vi "fgv_DO_q.vi"(7 "cmd":T1, 8 "error in":errorcluster, 11 "data":T2=enum."start") -> (0 "error out":errorcluster, 3 "queue out":refnum<queue>)   [LabVIEW 2019]
uses:
  _ctrl/start.ctl
  _ctrl/create-rw-close.ctl
  Durability/common/UI.ctl
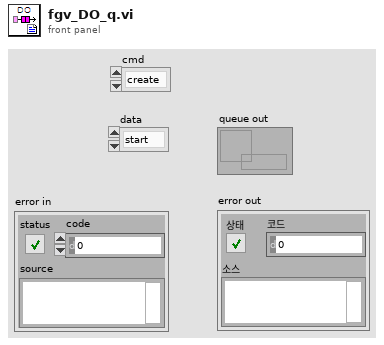
[diagram p1: front panel]
types:
  T1 = typedef "create-rw-close.ctl" = enum16{"create", "write", "read", "delete", "close"}
  T2 = typedef "start.ctl" = enum16{"init", "open", "set", "start", "stop", "read", "read_items", "query", "close", "T_single", "reset", "exit"}
  T3 = typedef "UI.ctl" = enum16{"Alarm yellow", "DL950 graph show", "DL950 graph clear", "AO value", "AO blink onoff", "Discharge relay", "Input Power", "Outpower", "Relay in1", "Relay in2", "Relay in3", "Relay in4", "Relay in5", "Relay in6", "Relay out1", "Relay out2", "Relay out3", "Relay out4", "Relay out5", "Relay out6", "Relay all off"}
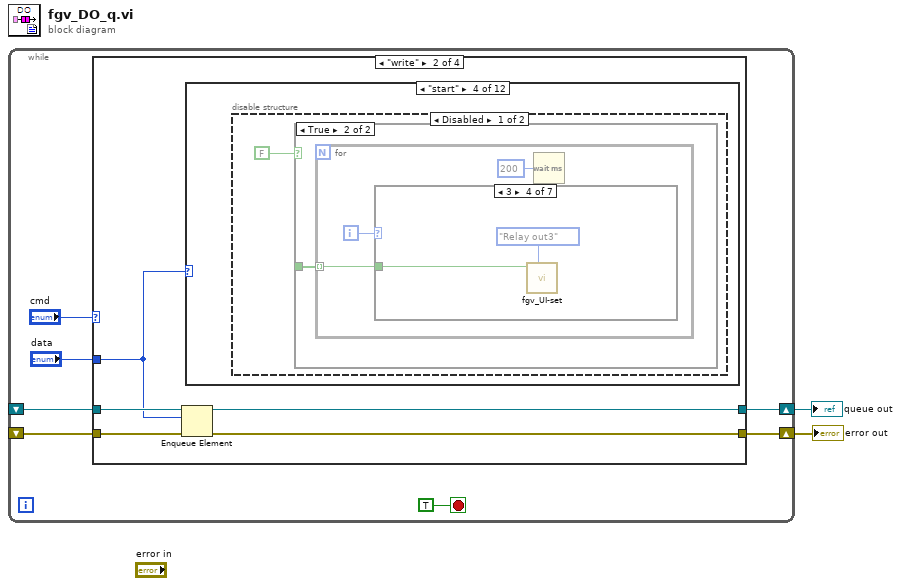
[diagram p0: block diagram]
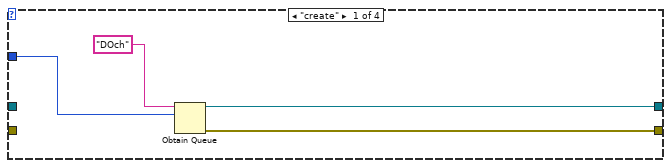
[diagram p2: hidden frame]
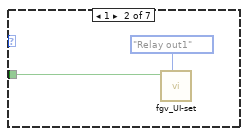
[diagram p8: hidden frame]
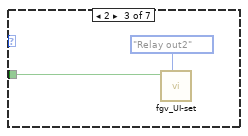
[diagram p9: hidden frame]
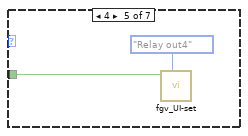
[diagram p10: hidden frame]
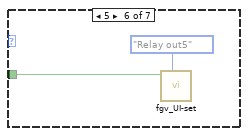
[diagram p11: hidden frame]
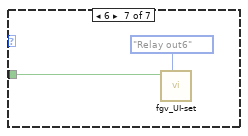
[diagram p12: hidden frame]
diagram:
  n1 = while {
    shift-right: [w6] -> w2
    shift-left: _ -> [w3]
    shift-right: [w5] -> w1
    shift-left: _ -> [w7]
    stop <- TRUE stop-if-true
    n2 = case shown="\"write\"" "cmd" {
      tunnel: w7 -> [_ w17 w36 _]
      tunnel: [w13 w16 w37 _] -> w6
      tunnel: [w12 w15 w36 _] -> w5
      tunnel: "data" -> [w10 w14 _ _]
      tunnel: w3 -> [_ w18 w37 w38]
      frame "create" {
        n3 = Obtain Queue(name (unnamed)="DOch" ("이름(이름없음)"), element data type=w10) -> (queue out=w13:refnum<queue>, error out=w12:errorcluster)  [unwired: 3 in, 1 out]
      }
      frame "write" {
        n4 = Enqueue Element(queue=w18, element=w14, error in (no error)=w17) -> (queue out=w16:refnum<queue>, error out=w15:errorcluster)  [unwired: 1 in, 1 out]
        n5 = case shown="\"start\"" w14 {
          frame "init", Default {
          }
          frame "open" {
          }
          frame "set" {
          }
          frame "start" {
            n6 = disable-structure shown="Disabled" {
              frame Disabled {
                n7 = case shown="True" FALSE {
                  tunnel: _ -> [_ w20]
                  frame False {
                  }
                  frame True {
                    n8 = for {
                      tunnel: w20 -> [w22] mode=indexing
                      i -> [w23]
                      n9 = case shown="3" w23 {
                        tunnel: w22 -> [_ w24 w26 w28 w30 w32 w34]
                        frame 0, Default {
                        }
                        frame 1 {
                          n10 = call "fgv_UI-set.vi"("cmd"=UI."Relay out1", "onoff"=w24) -> ()  [unwired: 9 in, 1 out]
                        }
                        frame 2 {
                          n11 = call "fgv_UI-set.vi"("cmd"=UI."Relay out2", "onoff"=w26) -> ()  [unwired: 9 in, 1 out]
                        }
                        frame 3 {
                          n12 = call "fgv_UI-set.vi"("cmd"=UI."Relay out3", "onoff"=w28) -> ()  [unwired: 9 in, 1 out]
                        }
                        frame 4 {
                          n13 = call "fgv_UI-set.vi"("cmd"=UI."Relay out4", "onoff"=w30) -> ()  [unwired: 9 in, 1 out]
                        }
                        frame 5 {
                          n14 = call "fgv_UI-set.vi"("cmd"=UI."Relay out5", "onoff"=w32) -> ()  [unwired: 9 in, 1 out]
                        }
                        frame 6 {
                          n15 = call "fgv_UI-set.vi"("cmd"=UI."Relay out6", "onoff"=w34) -> ()  [unwired: 9 in, 1 out]
                        }
                      }
                      n16 = Wait (ms)(milliseconds to wait=u32 200) -> ()  [unwired: 1 out]
                    }
                  }
                }
              }
              frame Enabled {
              }
            }
          }
          frame "stop" {
          }
          frame "read" {
          }
          frame "read_items" {
          }
          frame "query" {
          }
          frame "close" {
          }
          frame "T_single" {
          }
          frame "reset" {
          }
          frame "exit" {
          }
        }
      }
      frame "read" {
      }
      frame "close", Default {
        n17 = Release Queue(queue=w38) -> ()  [unwired: 2 in, 3 out]
      }
    }
  }
  "queue out" <- w2
  "error out" <- w1
